vi "TCP Multiple Connections - Client 1.vi"() -> ()   [LabVIEW 2018]
doc: "Establishes a connection to TCP Multiple Connections - Server.vi. After you click the Stop button, this VI sends a single character to tell the Server VI to terminate the connection."
panel:
  in  "Color Box":u32(colorbox)
  in  "Server Closed":string="The server VI closed the connection."
  out "Data from Server":dbl(graph)
  in  "Stop":bool
  # "Overview: Demonstrates the use of the TCP functions to connect to a TCP server VI that is sending data to multiple client VIs.\nInstructions:\n1. Ensure TCP Multiple Connections - Server.vi is already running.\n2. Run the VI.\n3. Note that the Data from Server chart starts updating, and the Number of Client Connections value on the server VI increments by 1.\n4. Click Stop to stop the VI. Note that the Number of Client Connections value on the server VI decrements by 1."
  # "1"
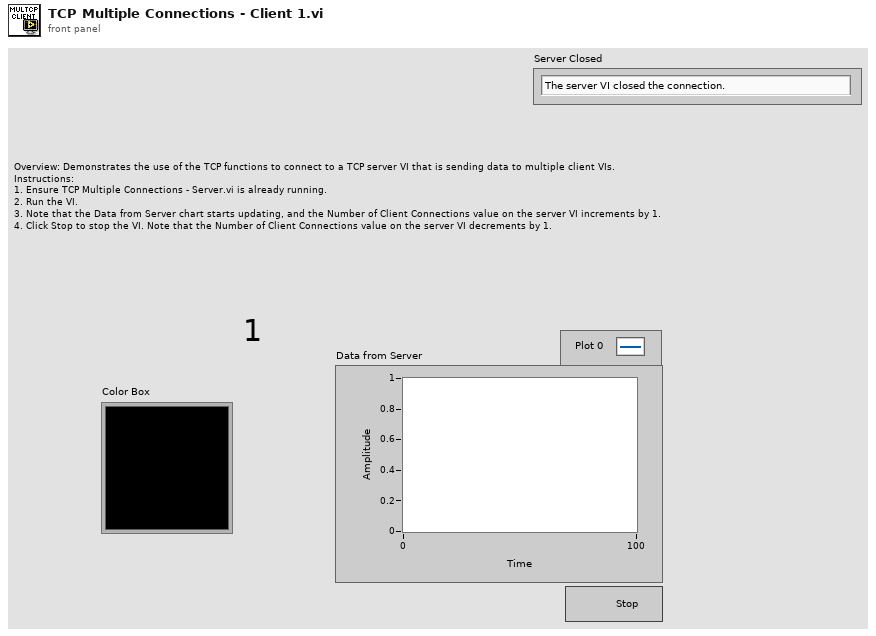
[diagram p1: front panel]
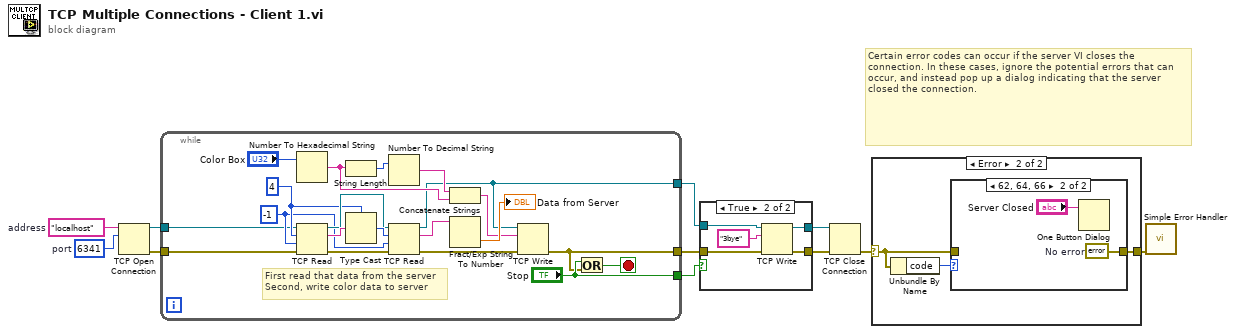
[diagram p0: block diagram]
diagram:
  w10 = u16 6341  # port
  w11 = "localhost"  # address
  # "Certain error codes can occur if the server VI closes the connection. In these cases, ignore the potential errors that can occur, and instead pop up a dialog indicating that the server closed the connection."
  n1 = TCP Open Connection(address=w11, remote port or service name=w10) -> (connection ID=w9:refnum<k5>, error out=w8:errorcluster)  [unwired: 1 in, 2 out]
  n2 = while {
    tunnel: ["Stop"] -> w3
    tunnel: [w15] -> w7
    tunnel: [w12] -> w5
    tunnel: w8 -> [w31]
    tunnel: w9 -> [w20]
    stop <- w26 stop-if-true
    w21 = -1
    w22 = 4
    # "First read that data from the server\nSecond, write color data to server"
    n3 = Number To Hexadecimal String(2:"Color Box") -> (0:w16:string)  [unwired: 1 in]
    n4 = TCP Read(connection ID=w20, bytes to read=w22, error in (no error)=w31, 9:w21) -> (connection ID out=w27:refnum<k5>, data out=w30:string, error out=w29:errorcluster)  [unwired: 1 out]
    n5 = String Length(string=w16) -> (length=w18:i32)
    n6 = Type Cast(type=w22, x=w30) -> (*(type *) &x=w28:i32)
    n7 = Number To Decimal String(number=w18) -> (decimal integer string=w17:string)  [unwired: 1 in]
    n8 = TCP Read(connection ID=w27, bytes to read=w28, error in (no error)=w29, 9:w21) -> (connection ID out=w15:refnum<k5>, data out=w24:string, error out=w13:errorcluster)  [unwired: 1 out]
    n9 = Concatenate Strings(w17, w16) -> (w14:string)
    n10 = Fract/Exp String To Number(string=w24) -> (number=→"Data from Server":dbl)  [unwired: 3 in, 1 out]
    n11 = TCP Write(connection ID=w15, data in=w14, error in (no error)=w13) -> (error out=w12:errorcluster)  [unwired: 1 in, 2 out]
    n12 = Or(x="Stop", y=w12) -> (x .or. y?=w26:bool)
  }
  n13 = case shown="True" w3 {
    tunnel: w7 -> [w33 w38]
    tunnel: [w33 w36] -> w6
    tunnel: w5 -> [w32 w37]
    tunnel: [w32 w35] -> w4
    frame False {
    }
    frame True {
      n14 = TCP Write(connection ID=w38, data in="3bye", error in (no error)=w37) -> (connection ID out=w36:refnum<k5>, error out=w35:errorcluster)  [unwired: 2 out]
    }
  }
  n15 = TCP Close Connection(connection ID=w6, error in (no error)=w4) -> (error out=w2:errorcluster)  [unwired: 2 out]
  n16 = case shown="Error" w2 {
    selector: w2 -> [w39 w41]
    tunnel: [w39 w40] -> w1
    frame No Error {
    }
    frame Error {
      n17 = Unbundle By Name(w41) -> ("code"=w42:i32)
      n18 = case shown="62, 64, 66" w42 {
        tunnel: w41 -> [w43 _]
        tunnel: [w43 w45] -> w40
        frame Default {
        }
        frame 62, 64, 66 {
          w45 = errorcluster {"status"=FALSE, "code"=0, "source"=""}  # No error
          n19 = One Button Dialog(message="Server Closed") -> ()  [unwired: 1 in, 1 out]
        }
      }
    }
  }
  n20 = call <vilib>:"Simple Error Handler.vi"("error in (no error)"=w1) -> ()  [unwired: 1 in, 8 out]
